vi "DraggingDresser-FINAL.vi"() -> ()   [LabVIEW 2014]
panel:
  out "Force":dbl[](array[numeric])
  out "Angle for Minimum Force":i32 format="%.1f"
  in  "Coefficient of Kinetic Friction":dbl format="%.1f"
  out "Waveform Graph":dbl[](graph)
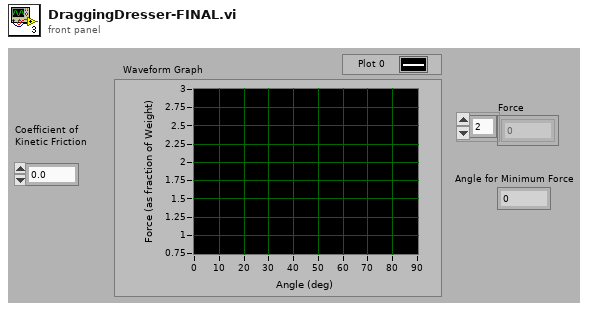
[diagram p1: front panel]
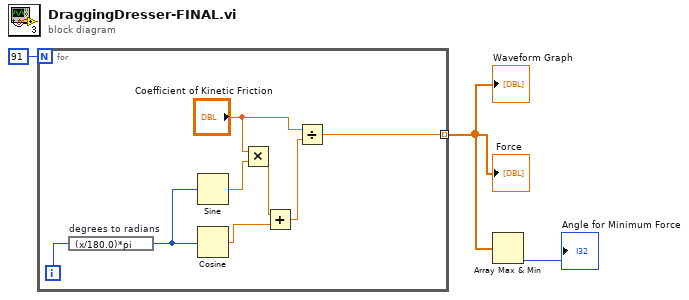
[diagram p0: block diagram]
diagram:
  n1 = for {
    N: 91 -> [_]
    tunnel: [w4] -> w3 mode=indexing
    i -> [w11]
    n2 = expression code="(x/180.0)*pi" "degrees to radians"(w11) -> (w10:i32)
    n3 = Sine(x=w10) -> (sin(x)=w9:dbl)
    n4 = Cosine(x=w10) -> (cos(x)=w8:dbl)
    n5 = Multiply(x="Coefficient of Kinetic Friction", y=w9) -> (x*y=w7:dbl)
    n6 = Add(x=w7, y=w8) -> (x+y=w5:dbl)
    n7 = Divide(x="Coefficient of Kinetic Friction", y=w5) -> (x/y=w4:dbl)
  }
  "Waveform Graph" <- w3
  "Force" <- w3
  n8 = Array Max & Min(array=w3) -> (min index (indices)=→"Angle for Minimum Force":i32)  [unwired: 3 out]
